vi "Request Message.vi"(4 "Activate Immediately? (T)":bool=TRUE, 5 "Return Priority (Normal)":T2=enum."Normal", 6 "Configured SubscriptionPolicy":refnum<class "ISubscriptionPolicy.lvclass">, 7 "Desired Notification Msg":refnum<class "Notification Msg.lvclass">, 8 "error in (no error)":errorcluster, 9 "Data Type":variant, 10 "Datum Name":string, 11 "IObserver in":refnum<class "IObserver.lvclass">) -> (0 "error out":errorcluster, 2 "Subscription Policy":T1, 3 "IObserver out":refnum<class "IObserver.lvclass">)   [LabVIEW 2020, in "IObserver.lvlib" / "IObserver.lvclass"]
doc: "<License>\nCopyright © 2017 Composed Systems, LLC | All rights reserved\nwww.composed.io\n\nAuthor: Ethan Stern <ethan.stern@composed.io>\n\nThis software is provided \"AS IS\" WITHOUT WARRANTIES, either express or implied, AND IS FOR EDUCATIONAL PURPOSES ONLY.\n</License>"
uses:
  <vilib>/gpm_packages/@cs/mva-core/Source/IObserver/IObserver/IObserver.lvclass
  C:/Program Files/National Instruments/LabVIEW 2020/vi.lib/ActorFramework/Actor/Actor.lvclass
  <vilib>/gpm_packages/@cs/transport/Source/Concrete/ActorMessageTransport/Notification Msg/Notification Msg.lvclass
  <vilib>/ActorFramework/Message Enqueuer/Message Priority.ctl
  <vilib>/gpm_packages/@cs/mva-core/Source/IMediator/ISubscriptionPolicy/ISubscriptionPolicy.lvclass
  <vilib>/gpm_packages/@cs/mva-core/Source/IMediator/ISubscriptionPolicy/ISubscriptionPolicy Reference.ctl
  <vilib>/ActorFramework/Actor/Actor.lvclass/Actor.ctl
  <vilib>/ActorFramework/Message Enqueuer/Message Enqueuer.lvclass/Message Enqueuer.ctl
  <vilib>/gpm_packages/@cs/transport/Source/Concrete/ActorMessageTransport/ActorMessageTransport.lvclass/ActorMessageTransport.ctl
  <vilib>/gpm_packages/@cs/mva-core/Source/IMediator/SubscriptionRequest/SubscriptionRequest.lvclass/SubscriptionRequest.ctl
  <vilib>/gpm_packages/@cs/mva-core/Source/IObserver/IObserver Messages/Subscribe Msg/Subscribe Msg.lvclass/Subscribe Msg.ctl
  <vilib>/ActorFramework/Message Enqueuer/Enqueue.vi
  <vilib>/ActorFramework/Message Enqueuer/Init from Existing Queue.vi
  <vilib>/ActorFramework/Message Enqueuer/Equals Not A Refnum.vi
  <vilib>/gpm_packages/@cs/transport/Source/Concrete/ActorMessageTransport/ActorMessageTransport.lvclass
  C:/Program Files/National Instruments/LabVIEW 2020/vi.lib/gpm_packages/@cs/transport/Source/ITransport/ITransport.lvclass
  <vilib>/gpm_packages/@cs/mva-core/Source/IObserver/IObserver Messages/Subscribe Msg/Subscribe Msg.lvclass
  C:/Program Files/National Instruments/LabVIEW 2020/vi.lib/ActorFramework/Message/Message.lvclass
  <vilib>/Utility/error.llb/Error Cluster From Error Code.vi
  <vilib>/ActorFramework/Message Priority Queue/Priority Enqueue.vi
  <vilib>/ActorFramework/Message Enqueuer/Message Enqueuer.lvclass
  <vilib>/gpm_packages/@cs/mva-core/Source/IMediator/SubscriptionRequest/SubscriptionRequest.lvclass
  <vilib>/ActorFramework/Actor/Actor.lvclass
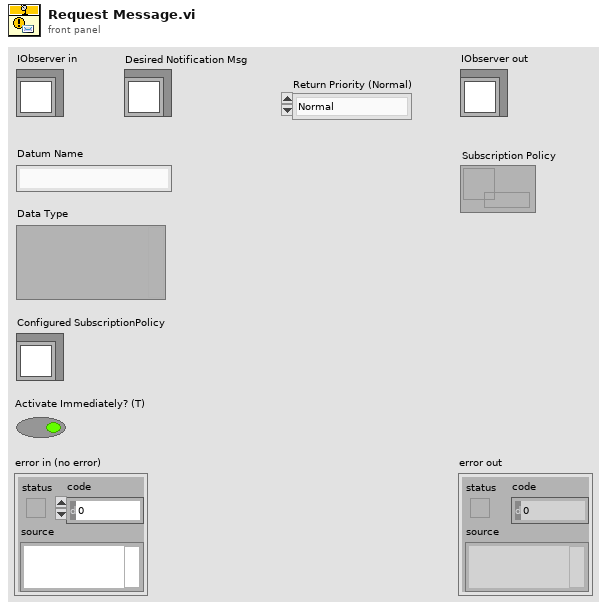
[diagram p1: front panel]
types:
  T1 = typedef "IMediator.lvlib/ISubscriptionPolicy.lvclass/ISubscriptionPolicy Reference.ctl" = refnum<data-value>
  T2 = typedef "Actor Framework.lvlib/Message Enqueuer.lvclass/Message Priority.ctl" = enum16{"Low", "Normal", "High"}
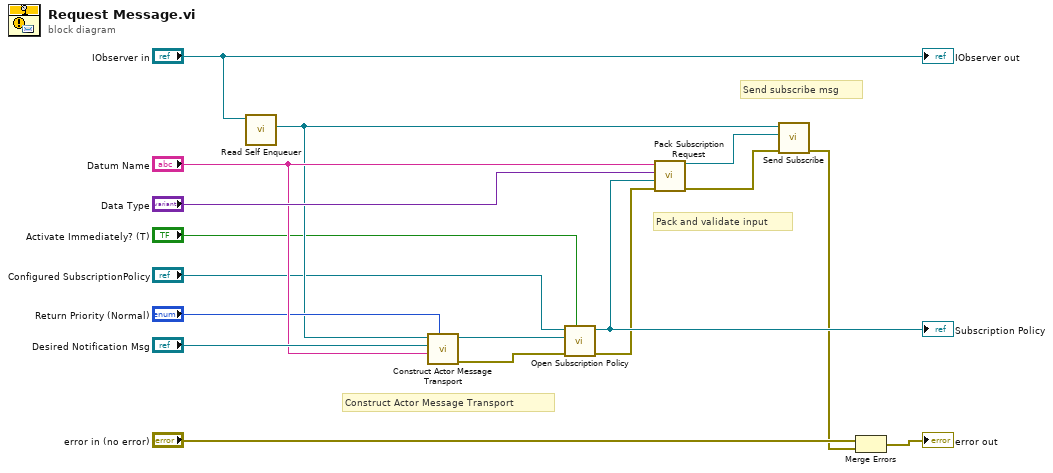
[diagram p0: block diagram]
diagram:
  # "Send subscribe msg"
  # "Pack and validate input"
  # "Construct Actor Message Transport"
  n1 = call <vilib>:"Read Self Enqueuer.vi"("Actor"="IObserver in") -> ("Self Enqueuer"=w8:refnum<class "Message Enqueuer.lvclass">)  [unwired: 10 in]
  n2 = call <vilib>:"Construct Actor Message Transport.vi"("Return Priority (Normal)"="Return Priority (Normal)", "Datum Name"="Datum Name", "Notification Msg"="Desired Notification Msg", "Message Enqueuer in"=w8) -> ("error out"=w7:errorcluster, "ActorMessageTransport"=w12:refnum<class "ActorMessageTransport.lvclass">)  [unwired: 6 in]
  n3 = call <vilib>:"Open Subscription Policy.vi"("Activate? (T)"="Activate Immediately? (T)", "error in (no error)"=w7, "Transport"=w12, "SubscriptionPolicy"="Configured SubscriptionPolicy") -> ("error out"=w3:errorcluster, "Subscription Policy"=w6:T1)  [unwired: 6 in]
  "Subscription Policy" <- w6
  n4 = call <vilib>:"Pack Subscription Request.vi"("error in (no error)"=w3, "Subscription Policy"=w6, "Type"="Data Type", "Datum Name"="Datum Name") -> ("error out"=w2:errorcluster, "SubscriptionRequest"=w16:refnum<class "SubscriptionRequest.lvclass">)  [unwired: 6 in]
  n5 = call <vilib>:"Send Subscribe.vi"("error in (no error)"=w2, "SubscriptionRequest"=w16, "Message Enqueuer"=w8) -> ("error out"=w1:errorcluster)  [unwired: 7 in, 1 out]
  n6 = Merge Errors("error in (no error)", w1) -> (→"error out":errorcluster)
  "IObserver out" <- "IObserver in"
